vi "TDMS_ Read-Write_into_File.vi"(4 "Channel Names to Read":string[](array[string]), 5 "Channel Names to Write":string[](array[string]), 6 "Number of Values in Raw Channel":u64, 7 "group name":string, 8 "Error in":errorcluster caption="Fehler (Eingang, kein Fehler)", 9 "Chennales to Process":T1, 10 "TDMS Write Files References":refnum<k34>[](array[refnum]), 11 "TDMS Raw-File Reference":refnum<k34>) -> (0 "Error out":errorcluster caption="Fehler (Ausgang)")   [LabVIEW 2016]
uses:
  Chennales to Process Custer.ctl
  File Progress Global.vi
  <vilib>/gmath/NI_Gmath.lvlib
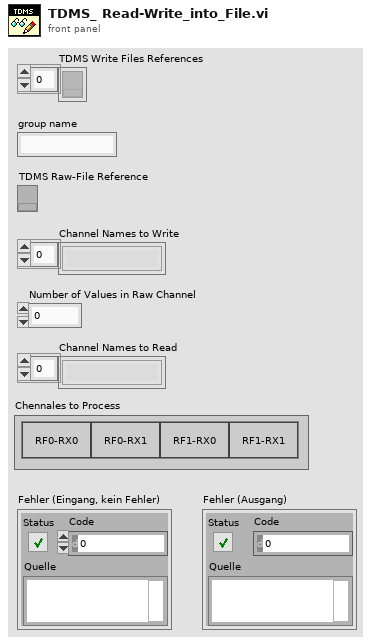
[diagram p1: front panel]
types:
  T1 = typedef "Chennales to Process Custer.ctl" = cluster{"RF0-RX0":bool, "RF0-RX1":bool, "RF1-RX0":bool, "RF1-RX1":bool}
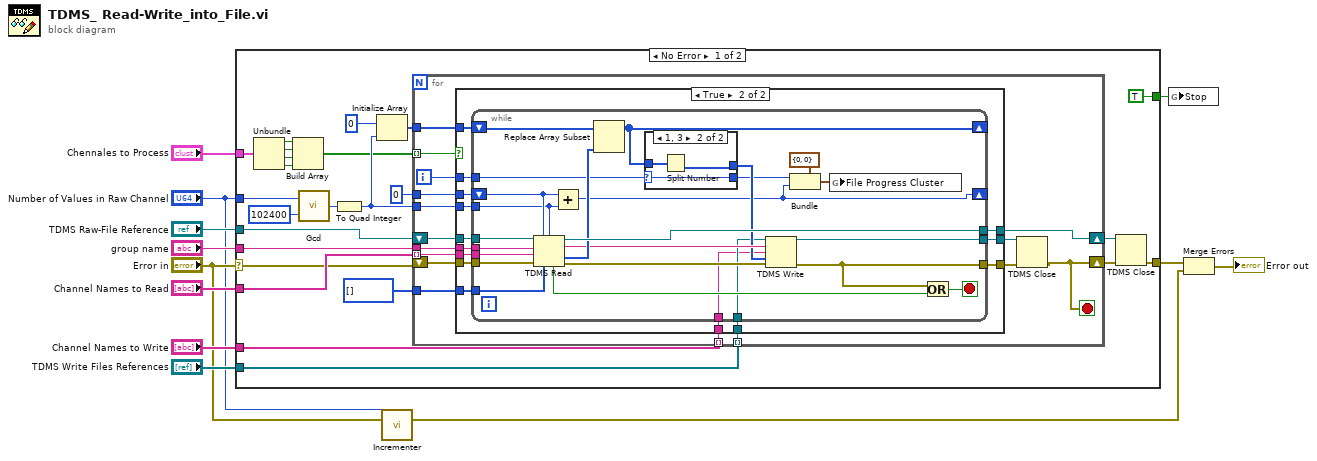
[diagram p0: block diagram]
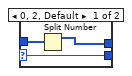
[diagram p3: hidden frame]
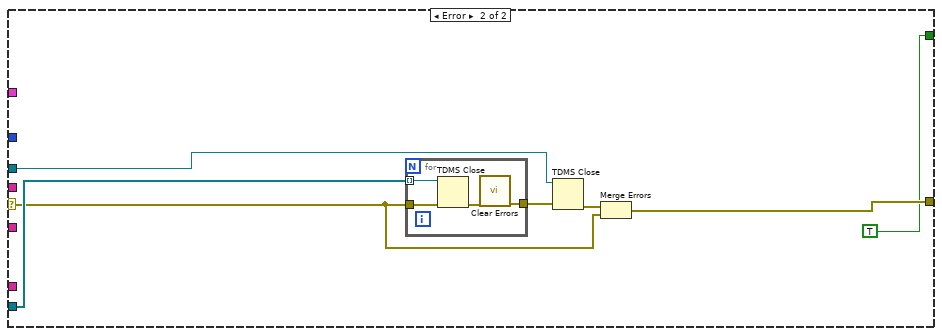
[diagram p4: hidden frame]
diagram:
  n1 = case shown="No Error" "Error in" {
    selector: "Error in" -> [w23 w103]
    tunnel: [w36 w102] -> w5
    tunnel: "Number of Values in Raw Channel" -> [w35 _]
    tunnel: "Channel Names to Write" -> [w33 _]
    tunnel: "Channel Names to Read" -> [w32 _]
    tunnel: "group name" -> [w29 _]
    tunnel: "TDMS Raw-File Reference" -> [w28 w105]
    tunnel: "TDMS Write Files References" -> [w24 w107]
    tunnel: [TRUE TRUE] -> w7
    tunnel: "Chennales to Process" -> [w18 _]
    frame No Error {
      n2 = Unbundle(w18) -> ("RF0-RX0"=w17:bool, "RF0-RX1"=w16:bool, "RF1-RX0"=w15:bool, "RF1-RX1"=w14:bool)
      n3 = Build Array(w17, w16, w15, w14) -> (w13:bool[])
      n4 = call <vilib>:"Gcd.vi"("y"=102400, "x"=w35) -> ("gcd(x,y)"=w21:i32)
      n5 = To Quad Integer(1:w21) -> (0:w20:i64)
      n6 = Initialize Array(u64 0 ("Numeric"), w20) -> (w26:u64[])
      n7 = for {
        tunnel: w24 -> [w52] mode=indexing
        tunnel: u64[] [] -> [w51]
        tunnel: w26 -> [w50]
        tunnel: i64 0 ("Numeric") -> [w49]
        tunnel: w20 -> [w48]
        tunnel: w29 -> [w45]
        shift-right: [w39] -> w30
        shift-left: w23 -> [w46]
        shift-right: [w44] -> w31
        shift-left: w28 -> [w47]
        tunnel: w32 -> [w43] mode=indexing
        tunnel: w33 -> [w42] mode=indexing
        tunnel: w13 -> [w37] mode=indexing
        i -> [w38]
        stop <- w39 stop-if-true
        n8 = case shown="True" w37 {
          tunnel: w52 -> [w54 w69]
          tunnel: w51 -> [_ w68]
          tunnel: w50 -> [_ w67]
          tunnel: w49 -> [_ w66]
          tunnel: w48 -> [_ w65]
          tunnel: w47 -> [w53 w64]
          tunnel: w46 -> [w55 w63]
          tunnel: w45 -> [_ w62]
          tunnel: [w53 w61] -> w44
          tunnel: w38 -> [_ w60]
          tunnel: w43 -> [_ w59]
          tunnel: w42 -> [_ w58]
          tunnel: [w55 w57] -> w41
          tunnel: [w54 w56] -> w40
          frame False {
          }
          frame True {
            n9 = while {
              tunnel: w64 -> [w94]
              tunnel: w63 -> [w93]
              tunnel: w69 -> [w77]
              tunnel: [w81] -> w57
              tunnel: [w92] -> w56
              tunnel: [w91] -> w61
              tunnel: w68 -> [w90]
              shift-right: [w87] -> _
              shift-left: w67 -> [w89]
              shift-right: [w71] -> _
              shift-left: w66 -> [w75]
              tunnel: w65 -> [w74]
              tunnel: w62 -> [w85]
              tunnel: w59 -> [w84]
              tunnel: w60 -> [w78]
              tunnel: w58 -> [w76]
              stop <- w82 stop-if-true
              n10 = TDMS Read(0:w94, 1:w75, 2:w74, 5:w85, 7:w84, 11:w93, 12:w90) -> (4:w91:refnum<k34>, 6:w83:string, 10:w88:u64[], 14:w80:bool, 15:w86:errorcluster)  [unwired: 1 in, 1 out]
              n11 = Add(x=w75, y=w74) -> (x+y=w71:i64)
              n12 = Replace Array Subset(array=w89, new element=w88) -> (w87:u64[])  [unwired: 1 in]
              n13 = case shown="1, 3" w78 {
                selector: w78 -> [w95 w98]
                tunnel: w87 -> [w97 w100]
                tunnel: [w96 w99] -> w79
                tunnel: [w95 w98] -> w70
                frame 0, 2, Default {
                  n14 = Split Number(x=w97) -> (hi(x)=w96:u32[])  [unwired: 1 out]
                }
                frame 1, 3 {
                  n15 = Split Number(x=w100) -> (lo(x)=w99:u32[])  [unwired: 1 out]
                }
              }
              n16 = TDMS Write(0:w77, 5:w83, 7:w76, 9:w79, 11:w86) -> (4:w92:refnum<k34>, 15:w81:errorcluster)  [unwired: 1 in, 2 out]
              n17 = Bundle(cluster=cluster{"Channel Count":i32, "Offset Count":i64} {"Channel Count"=0, "Offset Count"=0} ("File Progress Cluster"), "Channel Count"=w70, "Offset Count"=w71) -> (w73:cluster{"Channel Count":i32, "Offset Count":i64})
              n18 = global write "File Progress Global.vi" "File Progress Cluster"(w73) -> ()
              n19 = Or(x=w81, y=w80) -> (x .or. y?=w82:bool)
            }
          }
        }
        n20 = TDMS Close(8:w41, 11:w40) -> (0:w39:errorcluster)  [unwired: 1 out]
      }
      n21 = TDMS Close(8:w30, 11:w31) -> (0:w36:errorcluster)  [unwired: 1 out]
    }
    frame Error {
      n22 = for {
        tunnel: w103 -> [w111]
        tunnel: w107 -> [w110] mode=indexing
        tunnel: [w108] -> w106
        n23 = TDMS Close(8:w111, 11:w110) -> (0:w109:errorcluster)  [unwired: 1 out]
        n24 = call <vilib>:"Clear Errors.vi"("error in (no error)"=w109) -> ("error out"=w108:errorcluster)  [unwired: 5 in, 1 out]
      }
      n25 = TDMS Close(8:w106, 11:w105) -> (0:w104:errorcluster)  [unwired: 1 out]
      n26 = Merge Errors(w104, w103) -> (w102:errorcluster)
    }
  }
  n27 = call "Incrementer.vi"("N"="Number of Values in Raw Channel", "error in (no error)"="Error in") -> ("error out"=w3:errorcluster)  [unwired: 13 in]
  n28 = global write "File Progress Global.vi" "Stop"(w7) -> ()
  n29 = Merge Errors(w5, w3) -> (→"Error out":errorcluster)
